vi "Data32--Const.vi"() -> (3 "Data32 Command":string)   [LabVIEW 2017, in "Communications Library.lvlib"]
uses:
  Communications Library.lvlib
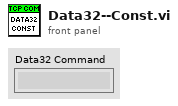
[diagram p1: front panel]
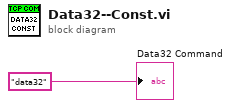
[diagram p0: block diagram]
diagram:
  "Data32 Command" <- "data32" ("data in")
